vi "ExCustomChip.vi"(1 "error in (no error)":errorcluster, 2 "Enable / Disable Custom Chip":bool=TRUE, 3 "Custom Chip Settings":T1={"Pre Y"=0, "Post Y"=0, "Parallel (Y) Size"=50, "Pre X"=0, "Post X"=0, "Seria (X) Size"=500}) -> (0 "error out":errorcluster)   [LabVIEW 2010]
uses:
  Open-Close Hardware/CamHandle.vi
panel:
  # "ExCustomChip.vi : this vi sets up the custom chip \nfeature of the Pixis camera."
  # "Vertical Dimension\nPre-Y + Parallel (Y)  Size + Post-Y"
  # "Horizontal Dimension\nPre-X + Serial (X)  Size + Post-X"
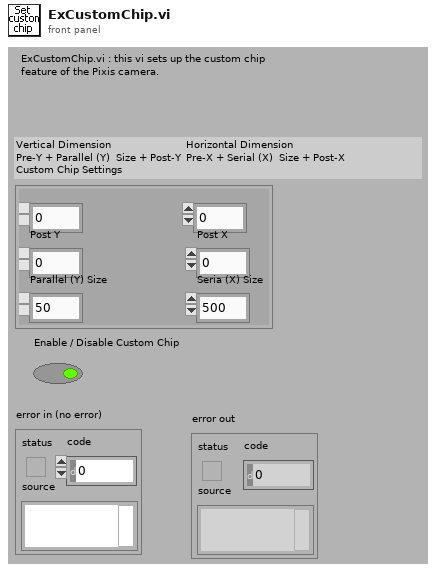
[diagram p1: front panel]
types:
  T1 = cluster{"Pre Y":u32, "Post Y":u32, "Parallel (Y) Size":u32, "Pre X":u32, "Post X":u32, "Seria (X) Size":u32}
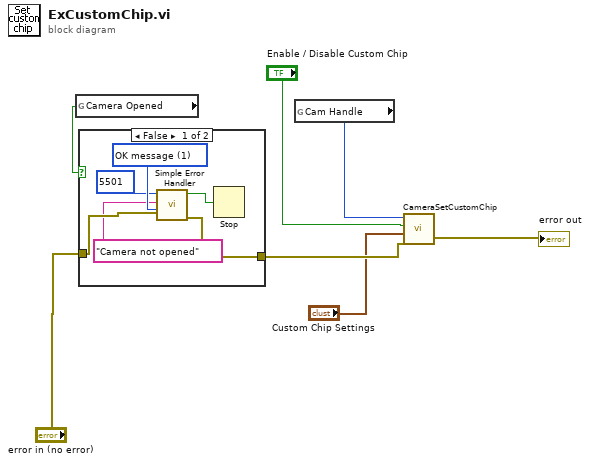
[diagram p0: block diagram]
diagram:
  n1 = global read "CamHandle.vi" "Camera Opened"() -> (w7:bool)
  n2 = case shown="False" w7 {
    tunnel: "error in (no error)" -> [w12 w14]
    tunnel: [w11 w14] -> w4
    frame False {
      w13 = u16 1 items=["no dialog", "OK message", "continue or stop message"] ("type of dialog (OK msg:1)")
      n3 = call <vilib>:"Simple Error Handler.vi"("error code (no error:0)"=5501, "error source (\" \")"="Camera not opened", "type of dialog (OK msg:1)"=w13, "error in (no error)"=w12) -> ("error?"=w9:bool, "error out"=w11:errorcluster)  [unwired: 1 in, 3 out]
      n4 = Stop(stop? (T)=w9) -> ()
    }
    frame True {
    }
  }
  n5 = global read "CamHandle.vi" "Cam Handle"() -> (w5:u32)
  n6 = call <userlib>:"CameraSetCustomChip.vi"("error in (no error)"=w4, "Custom Chip Settings"="Custom Chip Settings", "Enable/Disable Custom Chip"="Enable / Disable Custom Chip", "Camera Handle"=w5) -> ("error out"=→"error out":errorcluster)  [unwired: 1 out]
